vi "Calculate Zoom.vi"(9 "Player 2 Position":refnum<class "Vector 2D.lvclass">, 10 "Player 1 Position":refnum<class "Vector 2D.lvclass">, 11 "Camera in":refnum<class "Camera.lvclass">) -> (3 "Camera out":refnum<class "Camera.lvclass">)   [LabVIEW 2021, in "Camera.lvclass"]
uses:
  Camera.lvclass
  Re-use Libraries/Vector 2D/Vector 2D.lvclass
  Camera.lvclass/Camera.ctl
panel:
  out "Waveform Chart":sgl(graph)
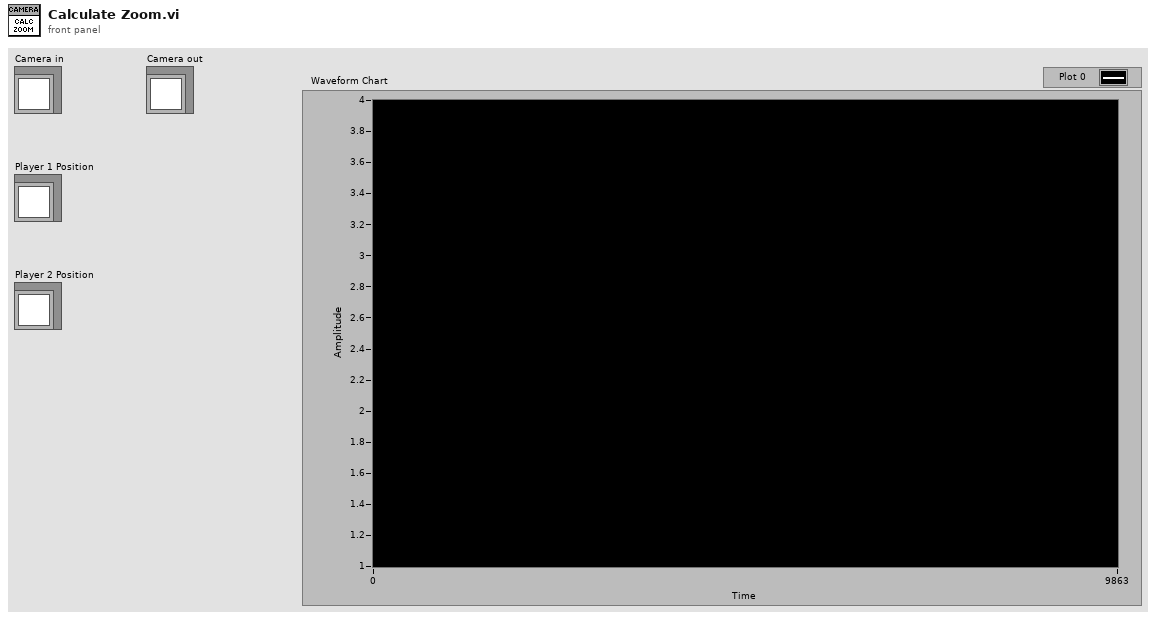
[diagram p1: front panel]
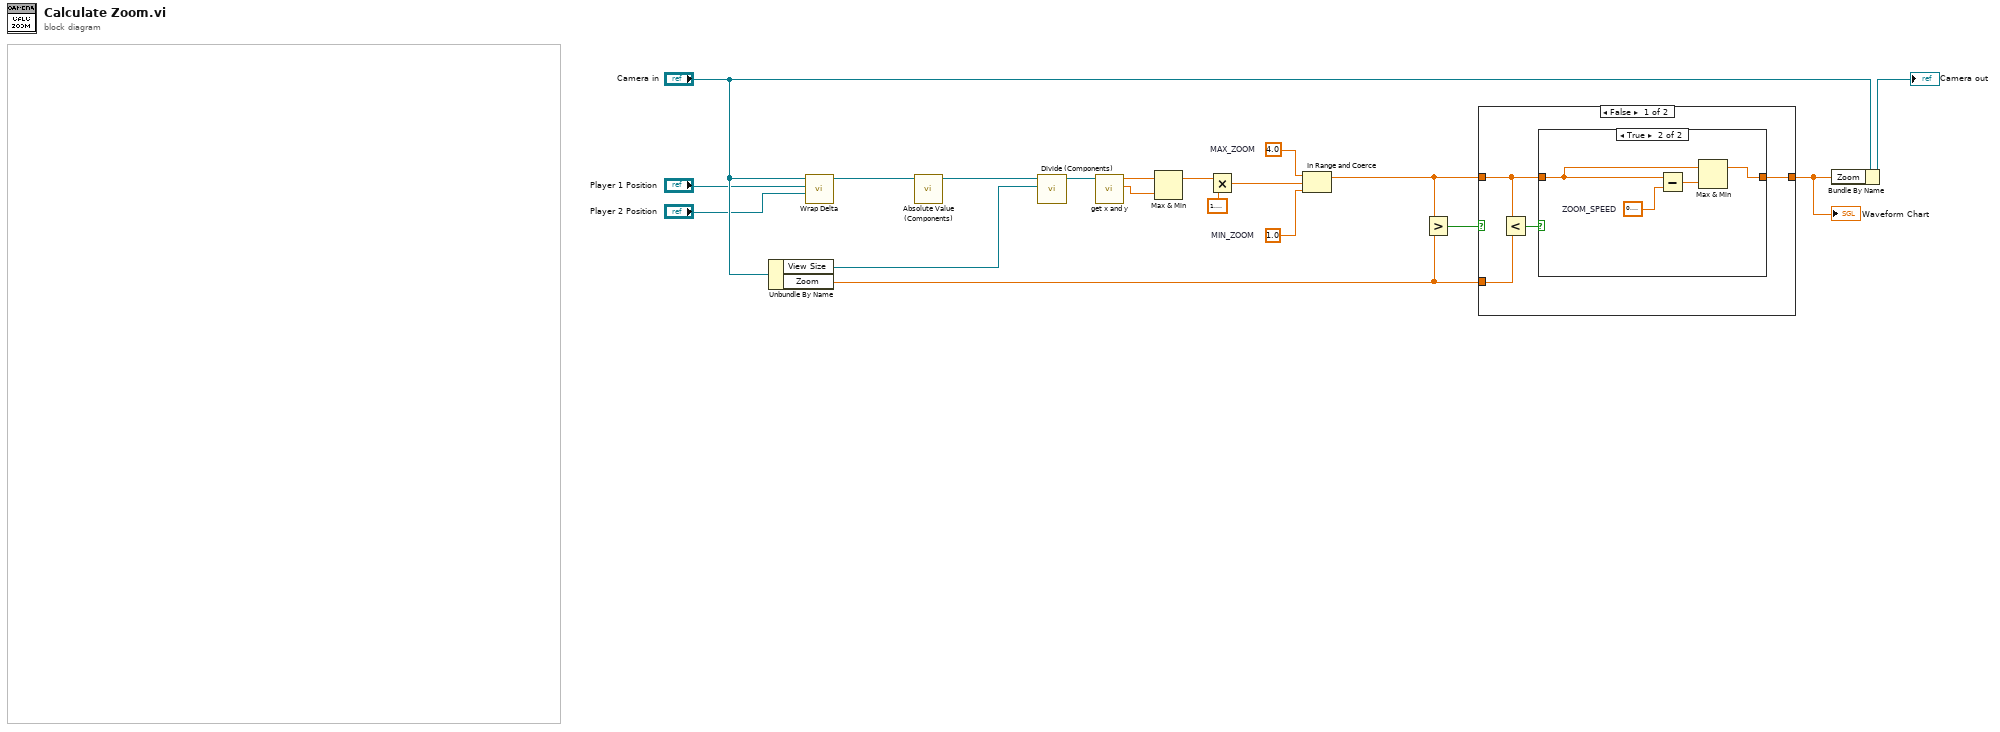
[diagram p0: block diagram]
diagram:
  w11 = sgl 1.0  # MIN_ZOOM
  w10 = sgl 4.0  # MAX_ZOOM
  n1 = Unbundle By Name("Camera in") -> ("View Size"=w14:refnum<class "Vector 2D.lvclass">, "Zoom"=w2:sgl)
  n2 = call "Wrap Delta.vi"("B"="Player 2 Position", "A"="Player 1 Position", "Camera in"="Camera in") -> ("Wrapped Delta"=w17:refnum<class "Vector 2D.lvclass">)  [unwired: 8 in]
  n3 = call "Absolute Value (Components).vi"("A"=w17) -> ("Absolute A"=w3:refnum<class "Vector 2D.lvclass">)  [unwired: 10 in]
  n4 = call "Divide (Components).vi"("B"=w14, "A"=w3) -> ("A+B"=w4:refnum<class "Vector 2D.lvclass">)  [unwired: 9 in]
  n5 = call "get x and y.vi"("Vector 2D in"=w4) -> ("y"=w6:sgl, "x"=w5:sgl)  [unwired: 9 in]
  n6 = Max & Min(x=w5, y=w6) -> (max(x,y)=w7:sgl)  [unwired: 1 out]
  n7 = Multiply(x=w7, y=sgl 1.2) -> (x*y=w9:sgl)
  n8 = In Range and Coerce(upper limit=w10, x=w9, lower limit=w11) -> (coerced(x)=w13:sgl)  [unwired: 1 out]
  n9 = Greater?(x=w13, y=w2) -> (0:w12:bool)
  n10 = case shown="False" w12 {
    tunnel: w13 -> [w21 w29]
    tunnel: [w20 w29] -> w1
    tunnel: w2 -> [w23 _]
    frame False {
      n11 = Less?(x=w21, y=w23) -> (x < y?=w22:bool)
      n12 = case shown="True" w22 {
        tunnel: w21 -> [w24 w26]
        tunnel: [w24 w27] -> w20
        frame False {
        }
        frame True {
          w28 = sgl 0.1  # ZOOM_SPEED
          n13 = Subtract(x=w26, y=w28) -> (x-y=w25:sgl)
          n14 = Max & Min(x=w26, y=w25) -> (max(x,y)=w27:sgl)  [unwired: 1 out]
        }
      }
    }
    frame True {
    }
  }
  "Waveform Chart" <- w1
  n15 = Bundle By Name(cluster="Camera in", "Zoom"=w1) -> (→"Camera out":refnum<class "Camera.lvclass">)
